vi "Write Line detector configuration.vi"(8 "error in (no error)":errorcluster, 10 "Configuration":T1={"Peak width guess"=0.0, "Background removal"=enum."NONE", "Smoothing"=enum."NONE", "Smooth window"=100.0, "Relative threshold"=0.0, "Finder algorithm"=enum."Basic", "Bgd window"=100.0, "Spectrum recorder module name"="Spectrum Recorder", "Fit window"=100.0, "Initial fit guess"=enum."Peak finder", "...with header "="", "Follow\npeaks"=FALSE, "Re-sample"=nan, "rusin\n.dat"=enum."NONE"} {"Re-sample" format="%#_6pHz"; "Fit window" format="%#_6pHz"; "Bgd window" format="%#_6pHz"; "Smooth window" format="%#_6pHz"; "Peak width guess" format="%#_6pHz"}, 11 "Line Detector in":refnum<class "Line Detector.lvclass">) -> (0 "error out":errorcluster, 3 "Line Detector out":refnum<class "Line Detector.lvclass">)   [LabVIEW 2016, in "Line Detector.lvclass"]
uses:
  Line Detector.lvclass
  C:/github/LabActor/Template Module/Template Module.lvclass
  Line Detector Configuration.ctl
  Template Module/Template Module.lvclass/Template Module.ctl
  Template Module/Write Configuration.vi
panel:
  # "Peak finder config"
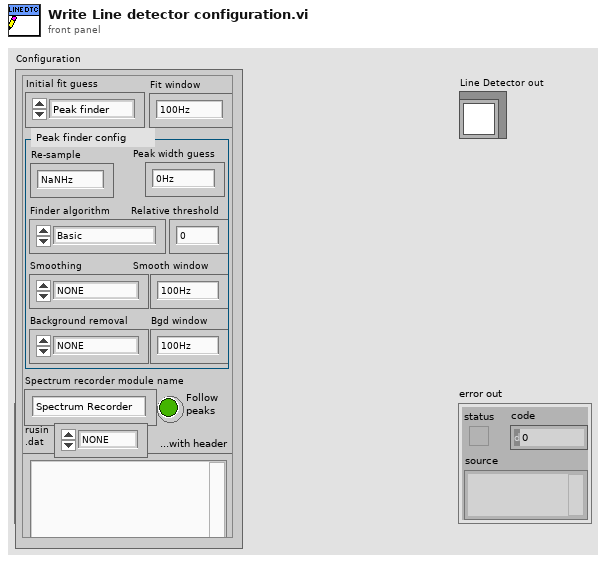
[diagram p1: front panel]
types:
  T1 = typedef "Line Detector Configuration.ctl" = cluster{"Peak width guess":dbl, "Background removal":enum16{"NONE", "High-pass", "Detrend"}, "Smoothing":enum16{"NONE", "Low-pass", "Denoise"}, "Smooth window":dbl, "Relative threshold":dbl, "Finder algorithm":enum16{"Basic", "Wavelet", "Wavelet+detrend"}, "Bgd window":dbl, "Spectrum recorder module name":string, "Fit window":dbl, "Initial fit guess":enum16{"Peak finder", "Last fit"}, "...with header ":string, "Follow\npeaks":bool, "Re-sample":dbl, "rusin\n.dat":enum16{"NONE", "DINES/cm2", "GPa"}}
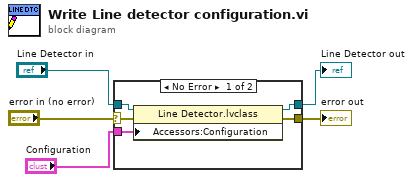
[diagram p0: block diagram]
diagram:
  n1 = case shown="No Error" "error in (no error)" {
    selector: "error in (no error)" -> [w10 w11]
    tunnel: [w9 w11] -> w4
    tunnel: [w7 w12] -> w2
    tunnel: "Line Detector in" -> [w8 w12]
    tunnel: "Configuration" -> [w6 _]
    frame No Error {
      n2 = property class="Line Detector.lvclass"(reference=w8, error in=w10, "Accessors:Configuration"=w6) -> (reference out=w7:refnum<class "Line Detector.lvclass">, error out=w9:errorcluster)
    }
    frame Error {
    }
  }
  "error out" <- w4
  "Line Detector out" <- w2
